vi "Load Category Instruments.vi"(8 "error in (no error)":errorcluster, 11 "Home in":refnum<class "Home.lvclass">) -> (0 "error out":errorcluster, 3 "Home out":refnum<class "Home.lvclass">)   [LabVIEW 2015, in "Category Library.lvlib" / "Home.lvclass"]
uses:
  Home.lvclass
  Settings Item/Settings.lvclass
  Welcome Item/Welcome.lvclass
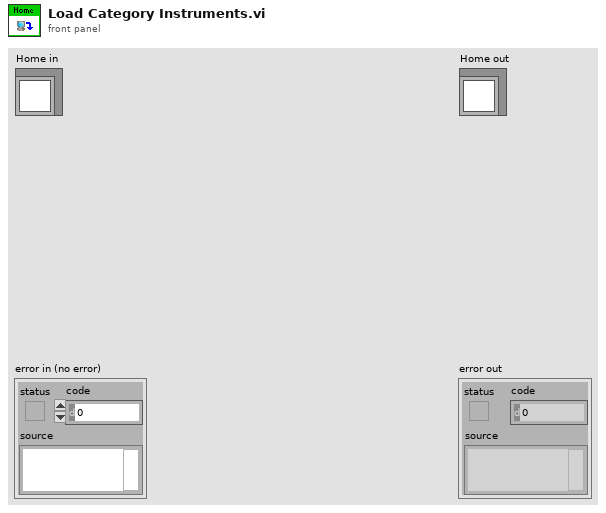
[diagram p1: front panel]
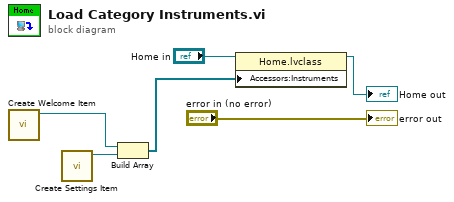
[diagram p0: block diagram]
diagram:
  n1 = call "Create Welcome Item.vi"() -> ("Welcome out"=w1:refnum<class "Welcome.lvclass">)  [unwired: 10 in, 1 out]
  n2 = call "Create Settings Item.vi"() -> ("Settings out"=w3:refnum<class "Settings.lvclass">)  [unwired: 10 in, 1 out]
  n3 = Build Array(w1, w3) -> (w2:refnum<class "Generic Item.lvclass">[])
  n4 = property class="Home.lvclass"(reference="Home in", "Accessors:Instruments"=w2) -> (reference out=→"Home out":refnum<class "Home.lvclass">)  [unwired: 1 in, 1 out]
  "error out" <- "error in (no error)"
